vi "BITMAPFILEHEADER.vi"(11 "Dimensions de l'image":i32[](array[numeric])) -> (3 "EN-TÊTE_FICHIER_BITMAP":u8[](array[numeric]))   [LabVIEW 2009]
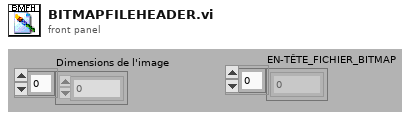
[diagram p1: front panel]
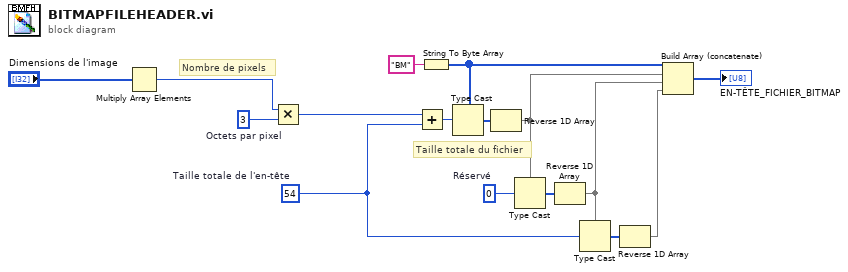
[diagram p0: block diagram]
diagram:
  w16 = 54  # Taille totale de l'en-tête
  w15 = 0  # Réservé
  w10 = 3  # Octets par pixel
  # "Taille totale du fichier"
  # "Nombre de pixels"
  n1 = Multiply Array Elements ("Multiplier les éléments du tableau")(1:"Dimensions de l'image") -> (0:w13:i32)
  n2 = Multiply ("Multiplier")(x=w13, y=w10) -> (x*y=w1:i32)
  n3 = Add ("Additionner")(x=w1, y=w16) -> (x+y=w8:i32)
  n4 = String To Byte Array ("Chaîne en tableau d'octets")(string="BM") -> (unsigned byte array=w9:u8[])
  n5 = Type Cast ("Adapter le type")(type=w9, x=w8) -> (*(type *) &x=w7:u8[])
  n6 = Reverse 1D Array ("Renverser un tableau 1D")(array=w7) -> (reversed array=w6:u8[])
  n7 = Type Cast ("Adapter le type")(type=w6, x=w15) -> (*(type *) &x=w5:u8[])
  n8 = Reverse 1D Array ("Renverser un tableau 1D")(array=w5) -> (reversed array=w4:u8[])
  n9 = Type Cast ("Adapter le type")(type=w4, x=w16) -> (*(type *) &x=w2:u8[])
  n10 = Reverse 1D Array ("Renverser un tableau 1D")(array=w2) -> (reversed array=w3:u8[])
  n11 = Build Array (concatenate) ("Construire un tableau")(w9, w6, w4, w3) -> (→"EN-TÊTE_FICHIER_BITMAP":u8[])
